vi "MM6.CheckStringMatch.vi"(10 "regular expression":string="TG[0-3]", 11 "string":string) -> (2 "exact match?":bool, 3 "string out":string)   [LabVIEW 2014, in "MM6.lvlib"]
doc: "This vi compares a textstring with a regular expression string and provides a boolean whether the strings match.\n\nauthor: Christopher Borgmann, christopher.borgmann@cern.ch"
uses:
  MM6.lvlib
panel:
  out "after substring":string
  out "length before":i32
  out "before substring":string
  out "length after":i32
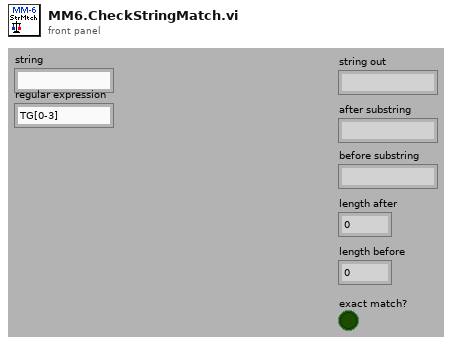
[diagram p1: front panel]
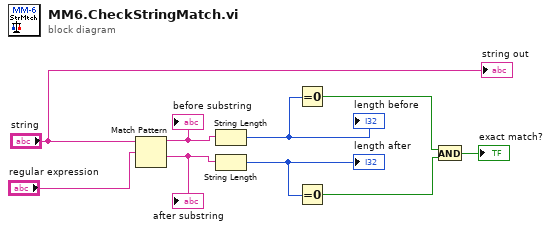
[diagram p0: block diagram]
diagram:
  n1 = Match Pattern(string="string", regular expression="regular expression") -> (before substring=w8:string, after substring=w9:string)  [unwired: 1 in, 2 out]
  "before substring" <- w8
  "after substring" <- w9
  n2 = String Length(string=w8) -> (length=w6:i32)
  "length before" <- w6
  n3 = String Length(string=w9) -> (length=w7:i32)
  "length after" <- w7
  n4 = Equal To 0?(x=w6) -> (x = 0?=w5:bool)
  n5 = Equal To 0?(x=w7) -> (x = 0?=w4:bool)
  n6 = And(x=w5, y=w4) -> (x .and. y?=→"exact match?":bool)
  "string out" <- "string"
